vi "WriteTravelUnitsRevolutions.vi"(8 "error in":errorcluster, 11 "VISA resource name":refnum<visa-resource-name>) -> (0 "error out":errorcluster, 3 "VISA resource name out":refnum<visa-resource-name>)   [LabVIEW 2019, in "Mark 10 TSTM-DC.lvlib"]
uses:
  Mark 10 TSTM-DC.lvlib
  Enum - TravelUnit.ctl
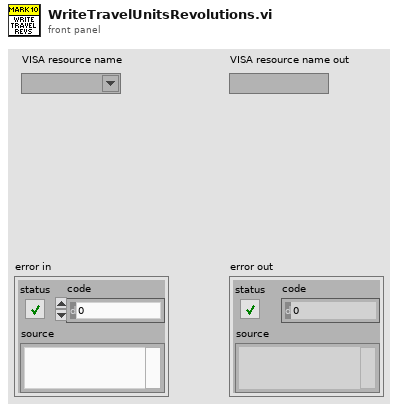
[diagram p1: front panel]
types:
  T1 = typedef "Mark 10 TSTM-DC.lvlib/Enum - TravelUnit.ctl" = enum16{"Revolutions", "Degrees"}
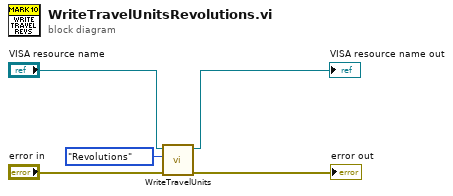
[diagram p0: block diagram]
diagram:
  n1 = call "WriteTravelUnits.vi"("error in"="error in", "TravelUnit"=Enum_-_TravelUnit."Revolutions", "VISA resource name"="VISA resource name") -> ("error out"=→"error out":errorcluster, "VISA resource name out"=→"VISA resource name out":refnum<visa-resource-name>)  [unwired: 7 in]
